vi "SngJntArmSim_UpdateX.vi"(8 "dT_Seconds":dbl=1.0, 9 "U":T4, 10 "current_xHat":T4, 11 "SINGLE_JOINT_ARM_SIM":T1 {"GearBox"."Kt_NMPerAmp" format="%13.5p"; "GearBox"."Kv_RadPerSecPerVolt" format="%13.5p"; "GearBox"."R_Ohms" format="%13.5p"; "GearBox"."FreeSpeed_RadPerSec" format="%13.5p"; "GearBox"."FreeCurrent_Amps" format="%13.5p"; "GearBox"."StallCurrent_Amps" format="%13.5p"; "GearBox"."StallTorque_NM" format="%13.5p"; "GearBox"."nominalVoltage_Volts" format="%13.5p"}) -> (3 "updated_xHat":T4)   [LabVIEW 2019, in "Trajectory_Library.lvlib"]
doc: "Creates a new LINEAR SYSTEM data cluster with the specified values. \n\n\nInputs: \n - XXX -- XXX.\n\nOutputs:\n - XXX -- XXX."
uses:
  Trajectory_Library.lvlib
  <vilib>/Analysis/Matrix/Datatypes/RealMatrix.ctl
  SINGLE_JOINT_ARM_SIM.ctl
  LINEAR_SYSTEM_SIM.ctl
  LINEAR_SYSTEM.ctl
  DCMOTOR.CTL
  MatBuilder_Create.vi
  <vilib>/Analysis/Matrix/NI_Matrix.lvlib
panel:
  # "<States, 1>"
  # "<Outputs, 1>"
  # "<Inputs, 1>"
  # "<Outputs, 1>"
  # "<States,States>"
  # "<States,Inputs>"
  # "<Outputs,States>"
  # "<Outputs,Inputs>"
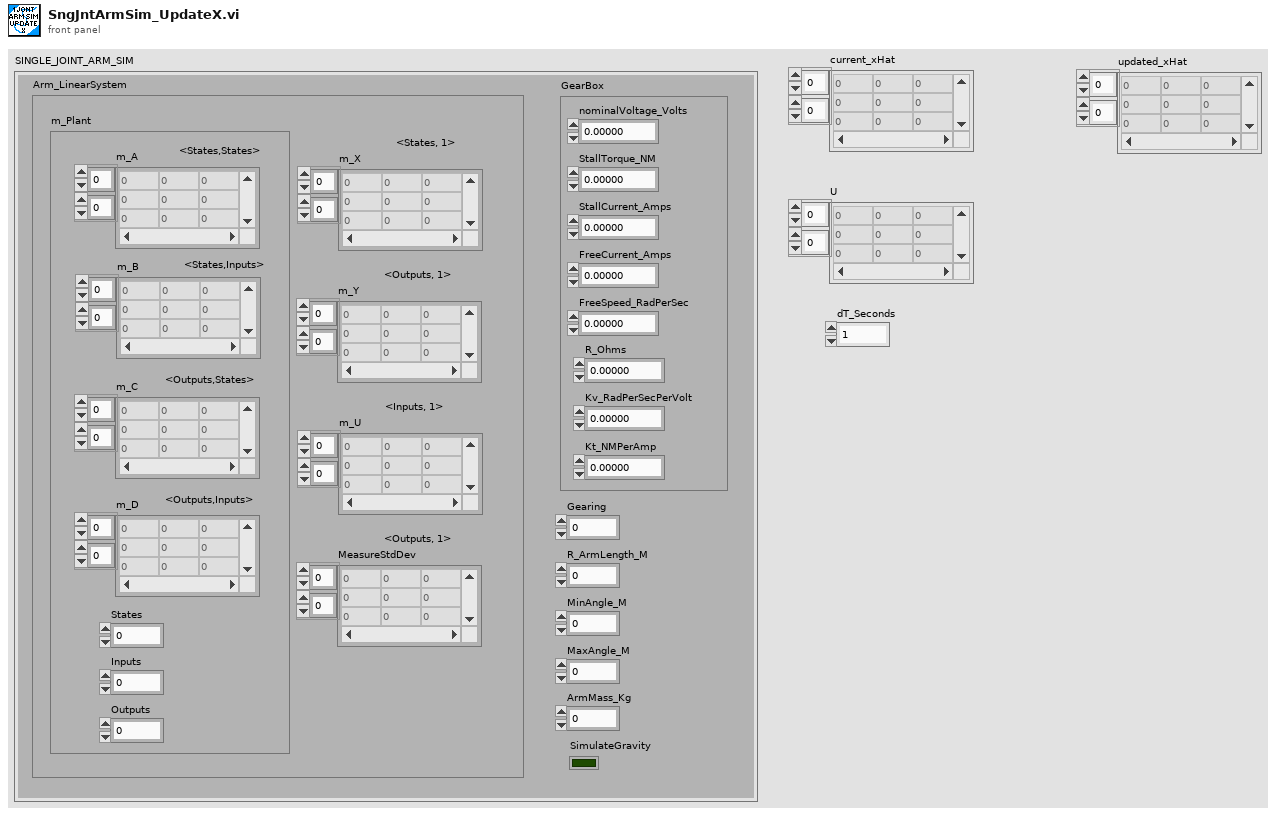
[diagram p1: front panel]
types:
  T1 = typedef "Trajectory_Library.lvlib/SINGLE_JOINT_ARM_SIM.ctl" = cluster{"Arm_LinearSystem":T2, "GearBox":T5, "Gearing":dbl, "R_ArmLength_M":dbl, "MinAngle_M":dbl, "MaxAngle_M":dbl, "ArmMass_Kg":dbl, "SimulateGravity":bool}
  T2 = typedef "Trajectory_Library.lvlib/LINEAR_SYSTEM_SIM.ctl" = cluster{"m_Plant":T3, "m_X":T4, "m_Y":T4, "m_U":T4, "MeasureStdDev":T4}
  T3 = typedef "Trajectory_Library.lvlib/LINEAR_SYSTEM.ctl" = cluster{"m_A":T4, "m_B":T4, "m_C":T4, "m_D":T4, "States":i32, "Inputs":i32, "Outputs":i32}
  T4 = typedef "NI_Matrix.lvlib/RealMatrix.ctl" = dbl[][]
  T5 = typedef "Trajectory_Library.lvlib/DCMOTOR.CTL" = cluster{"nominalVoltage_Volts":dbl, "StallTorque_NM":dbl, "StallCurrent_Amps":dbl, "FreeCurrent_Amps":dbl, "FreeSpeed_RadPerSec":dbl, "R_Ohms":dbl, "Kv_RadPerSecPerVolt":dbl, "Kt_NMPerAmp":dbl}
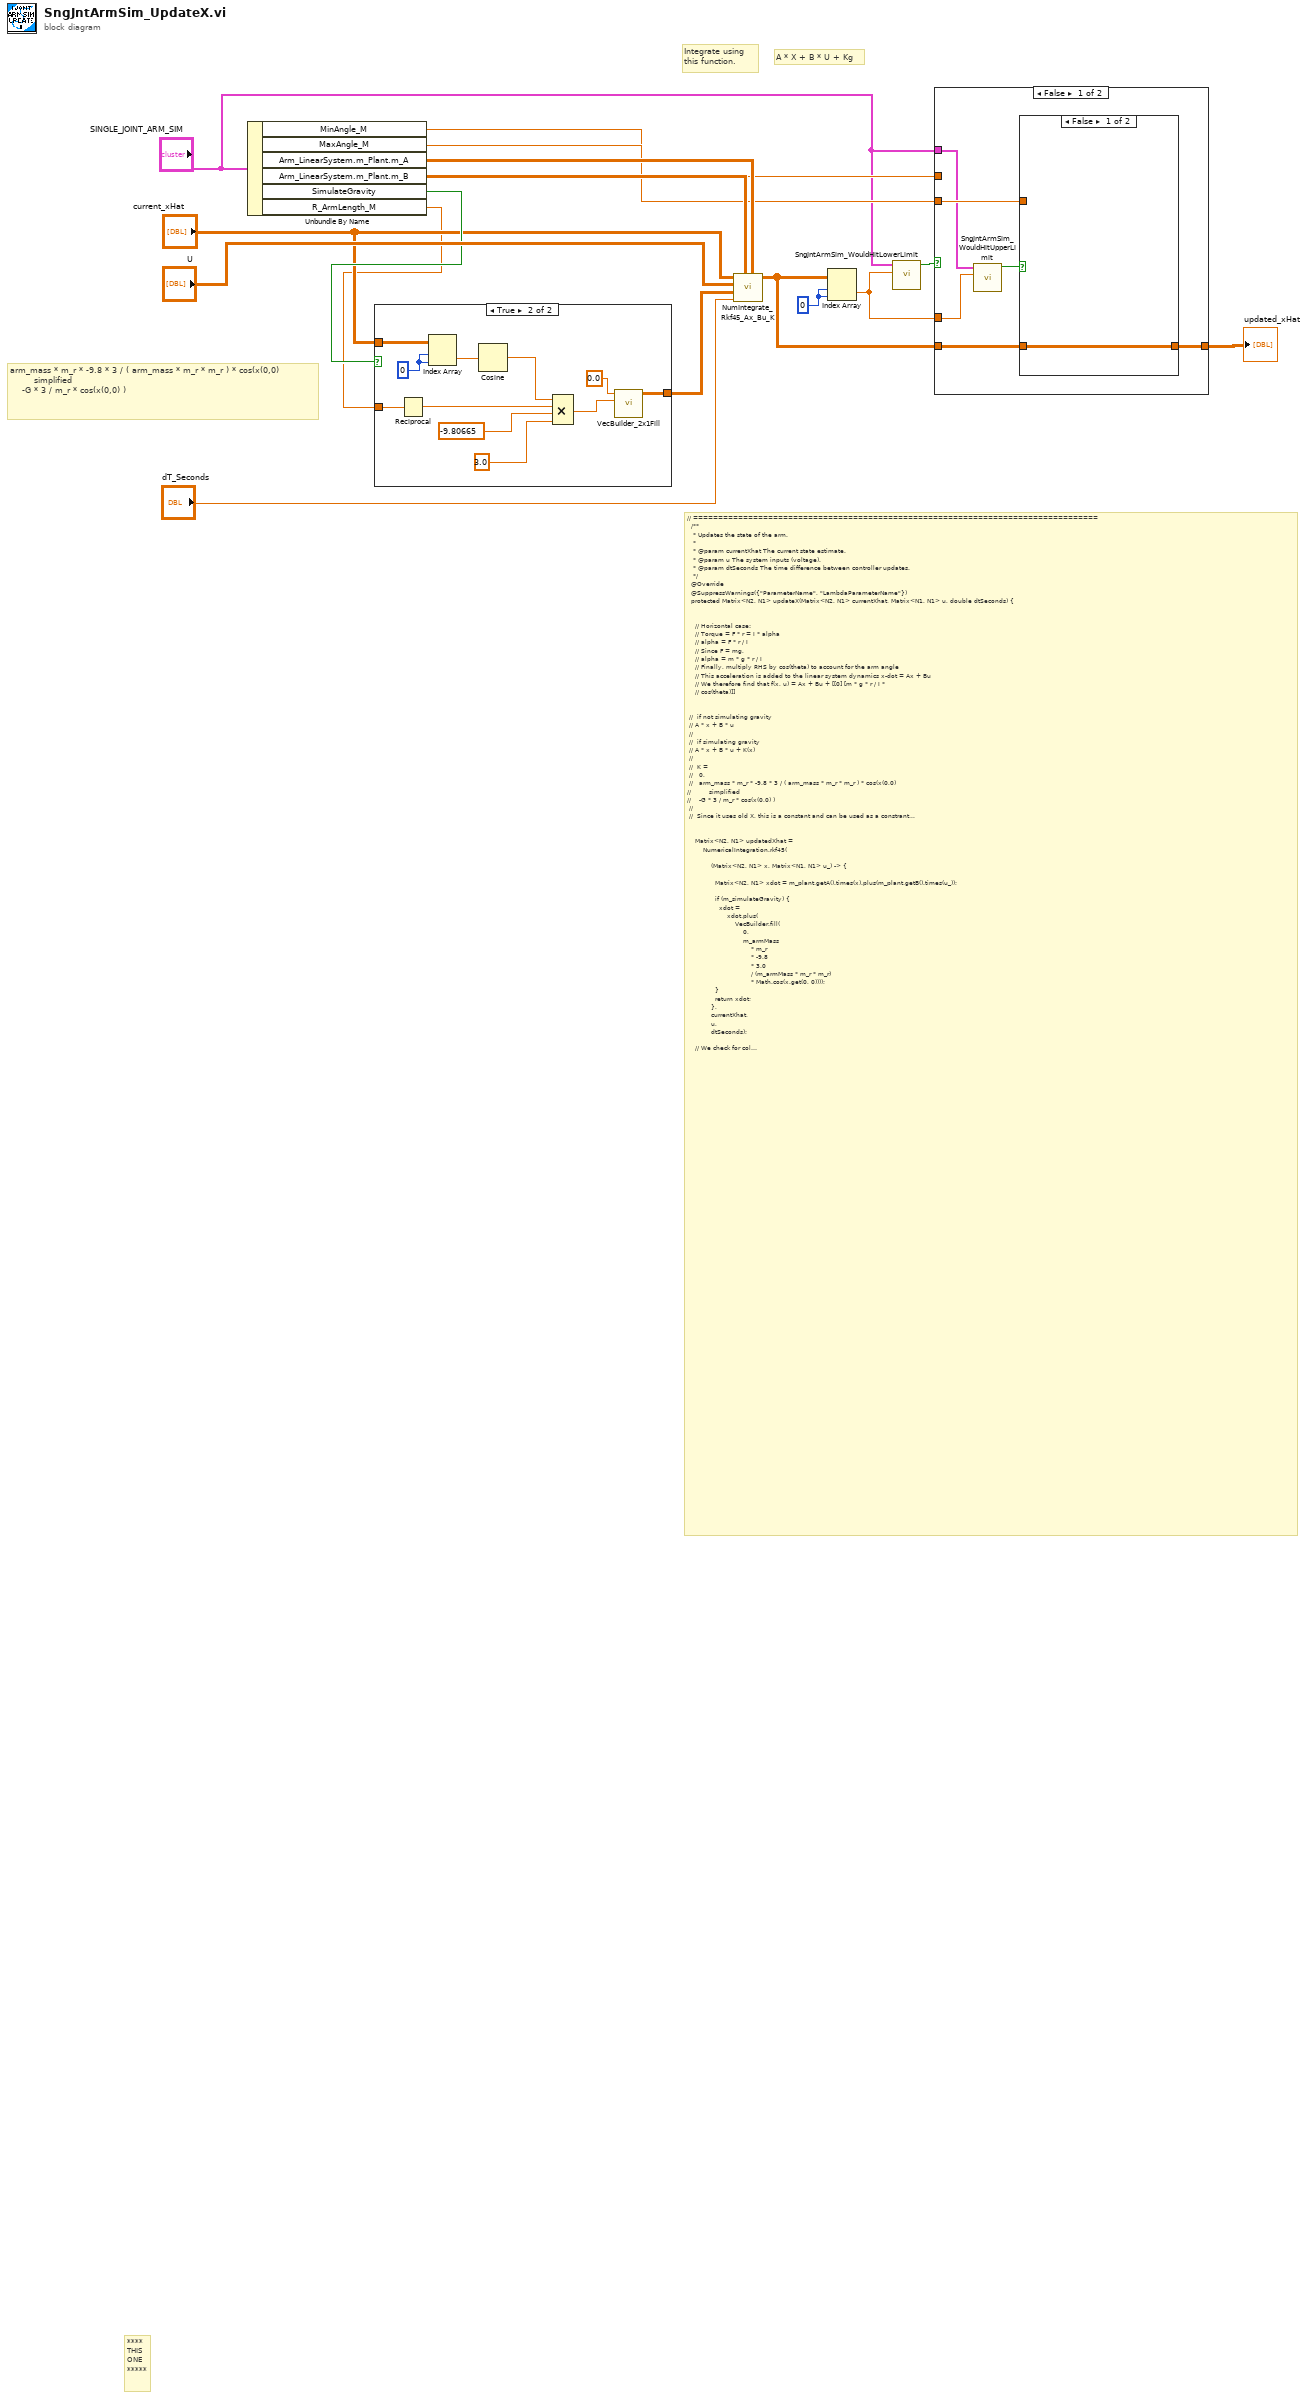
[diagram p0: block diagram]
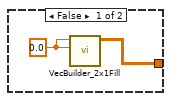
[diagram p2: hidden frame]
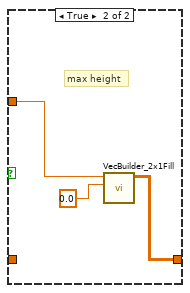
[diagram p3: hidden frame]
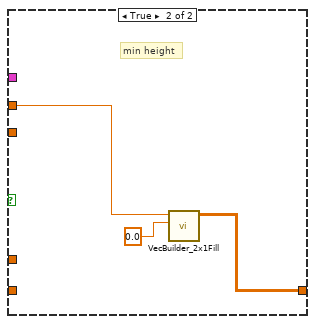
[diagram p4: hidden frame]
diagram:
  w11 = 0 ("index (row)")
  # "arm_mass * m_r * -9.8 * 3 / ( arm_mass * m_r * m_r ) * cos(x(0,0)\n        simplified\n    -G * 3 / m_r * cos(x(0,0) )"
  # "Integrate using\nthis function."
  # "A * X + B * U + Kg"
  # "// =================================================================================\n  /**\n   * Updates the state of the arm.\n   *\n   * @param currentXhat The current state estimate.\n   * @param u The system inputs (voltage).\n   * @param dtSeconds The time difference between controller updates.\n   */\n  @Override\n  @SuppressWarnings({\"ParameterName\", \"LambdaParameterName\"})\n  protected Matrix<N2, N1> updateX(Matrix<N2, N1> currentXhat, Matrix<N1, N1> u, double dtSeconds) {\n\n\n    // Horizontal case:\n    // Torque = F * r = I * alpha\n    // alpha = F * r / I\n    // Since F = mg,\n    // alpha = m * g * r / I\n    // Finally, multiply RHS by cos(theta) to account for the arm angle\n    // This acceleration is added to the linear system dynamics x-dot = Ax + Bu\n    // We therefore find that f(x, u) = Ax + Bu + [[0] [m * g * r / I *\n    // cos(theta)]]\n\n\n\t//  if not simulating gravity\n\t//\tA * x + B * u\n\t//\n\t//  if simulating gravity\n\t//\tA * x + B * u + K(x)\n\t//\n\t//\t\tK =\n\t//\t\t\t0,\n\t//\t\t\tarm_mass * m_r * -9.8 * 3 / ( arm_mass * m_r * m_r ) * cos(x(0,0)\n//         simplified\n//    -G * 3 / m_r * cos(x(0,0) )\n\t//\t\n\t//\t\tSince it uses old X, this is a constant and can be used as a constrant...\t\n\n\n    Matrix<N2, N1> updatedXhat =\n        NumericalIntegration.rkf45(\n\n            (Matrix<N2, N1> x, Matrix<N1, N1> u_) -> {\n\n              Matrix<N2, N1> xdot = m_plant.getA().times(x).plus(m_plant.getB().times(u_));\n\n              if (m_simulateGravity) {\n                xdot =\n                    xdot.plus(\n                        VecBuilder.fill(\n                            0,\n                            m_armMass\n                                * m_r\n                                * -9.8\n                                * 3.0\n                                / (m_armMass * m_r * m_r)\n                                * Math.cos(x.get(0, 0))));\n              }\n              return xdot;\n            },\n            currentXhat,\n            u,\n            dtSeconds);\n\n    // We check for collision after updating xhat\n    if (wouldHitLowerLimit(updatedXhat.get(0, 0))) {\n      return VecBuilder.fill(m_minAngle, 0);\n    }\n    if (wouldHitUpperLimit(updatedXhat.get(0, 0))) {\n      return VecBuilder.fill(m_maxAngle, 0);\n    }\n    return updatedXhat;\n  }"
  # "****\nTHIS\nONE\n*****"
  n1 = Unbundle By Name("SINGLE_JOINT_ARM_SIM") -> ("MinAngle_M"=w5:dbl, "MaxAngle_M"=w10:dbl, "Arm_LinearSystem.m_Plant.m_A"=w16:T4, "Arm_LinearSystem.m_Plant.m_B"=w15:T4, "SimulateGravity"=w3:bool, "R_ArmLength_M"=w1:dbl)
  n2 = case shown="True" w3 {
    tunnel: [w17 w28] -> w13
    tunnel: "current_xHat" -> [_ w26]
    tunnel: w1 -> [_ w24]
    frame False {
      w18 = 0.0 ("R0")
      n3 = call "VecBuilder_2x1Fill.vi"("R1"=w18, "R0"=w18) -> ("output matrix"=w17:T4)  [unwired: 9 in]
    }
    frame True {
      w27 = 0 ("index (row)")
      n4 = Reciprocal(x=w24) -> (1/x=w22:dbl)
      n5 = Index Array(array=w26, index (row)=w27, index (col)=w27) -> (element=w25:dbl)
      n6 = Cosine(x=w25) -> (cos(x)=w23:dbl)
      n7 = Compound Arithmetic op=MULTIPLY(w23, w22, -9.80665 ("R1"), 3.0 ("R1")) -> (w19:dbl)
      n8 = call "VecBuilder_2x1Fill.vi"("R1"=w19, "R0"=0.0) -> ("output matrix"=w28:T4)  [unwired: 9 in]
    }
  }
  n9 = call "NumIntegrate_Rkf45_Ax_Bu_K.vi"("A"=w16, "B"=w15, "dT_Seconds"="dT_Seconds", "K"=w13, "U"="U", "X"="current_xHat") -> ("Return X"=w9:T4)  [unwired: 4 in, 1 out]
  n10 = Index Array(array=w9, index (row)=w11, index (col)=w11) -> (element=w6:dbl)
  n11 = call "SngJntArmSim_WouldHitLowerLimit.vi"("Angle_Rads"=w6, "SingleJointArmSim"="SINGLE_JOINT_ARM_SIM") -> ("WouldHitLowLimit"=w7:bool)  [unwired: 9 in]
  n12 = case shown="False" w7 {
    tunnel: w10 -> [w31 _]
    tunnel: w9 -> [w35 _]
    tunnel: [w34 w40] -> w8
    tunnel: w6 -> [w32 _]
    tunnel: w5 -> [_ w41]
    tunnel: "SINGLE_JOINT_ARM_SIM" -> [w30 _]
    frame False {
      n13 = call "SngJntArmSim_WouldHitUpperLimit.vi"("Angle_Rad"=w32, "SingleJointArmSim"=w30) -> ("Would Hit HIgh LImit"=w33:bool)  [unwired: 9 in]
      n14 = case shown="False" w33 {
        tunnel: w35 -> [w36 _]
        tunnel: [w36 w37] -> w34
        tunnel: w31 -> [_ w38]
        frame False {
        }
        frame True {
          # "max height"
          n15 = call "VecBuilder_2x1Fill.vi"("R1"=0.0, "R0"=w38) -> ("output matrix"=w37:T4)  [unwired: 9 in]
        }
      }
    }
    frame True {
      # "min height"
      n16 = call "VecBuilder_2x1Fill.vi"("R1"=0.0, "R0"=w41) -> ("output matrix"=w40:T4)  [unwired: 9 in]
    }
  }
  "updated_xHat" <- w8
